vi "Write Locations DVR.vi"(8 "error in (no error)":errorcluster, 10 "Locations DVR":refnum<data-value>, 11 "Picture in":refnum<class "Picture.lvclass">) -> (0 "error out":errorcluster, 3 "Picture out":refnum<class "Picture.lvclass">)   [LabVIEW 2015, in "Picture.lvclass"]
uses:
  Picture.lvclass
  Picture.lvclass/Picture.ctl
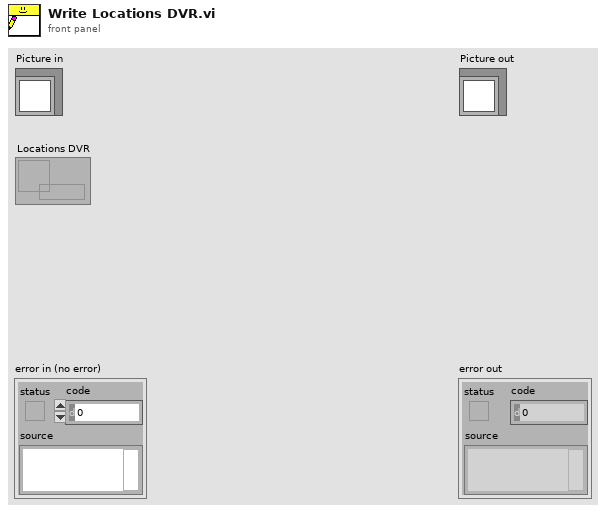
[diagram p1: front panel]
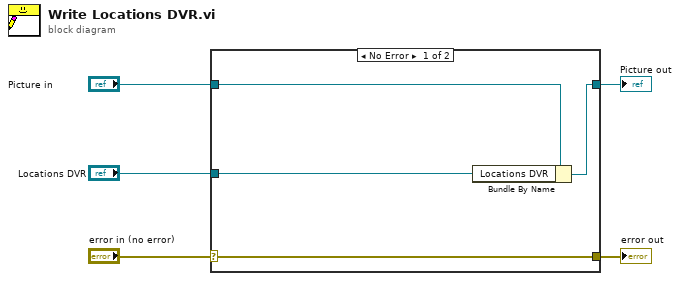
[diagram p0: block diagram]
diagram:
  n1 = case shown="No Error" "error in (no error)" {
    selector: "error in (no error)" -> [w9 w10]
    tunnel: [w9 w10] -> w4
    tunnel: [w7 w11] -> w2
    tunnel: "Picture in" -> [w8 w11]
    tunnel: "Locations DVR" -> [w6 _]
    frame No Error {
      n2 = Bundle By Name(cluster=w8, "Locations DVR"=w6) -> (w7:refnum<class "Picture.lvclass">)
    }
    frame Error {
    }
  }
  "error out" <- w4
  "Picture out" <- w2
